vi "Add to Symbol Map.vi"(8 "error in (no error)":errorcluster, 9 ".NET Symbol Information":refnum<k24>, 10 "Symbol Name":string, 11 "TwinCAT ADS in":refnum<class "TwinCAT ADS.lvclass">) -> (0 "error out":errorcluster, 2 "Success?":bool, 3 "TwinCAT ADS out":refnum<class "TwinCAT ADS.lvclass">)   [LabVIEW 2018, in "TwinCAT ADS.lvclass"]
uses:
  TwinCAT ADS.lvclass
  TwinCAT.Ads
  TwinCAT ADS.lvclass/TwinCAT ADS.ctl
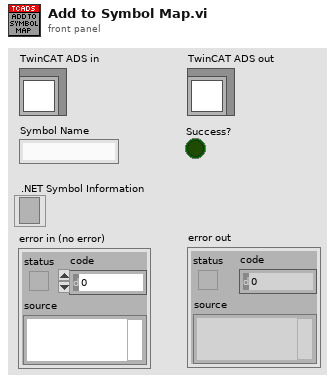
[diagram p1: front panel]
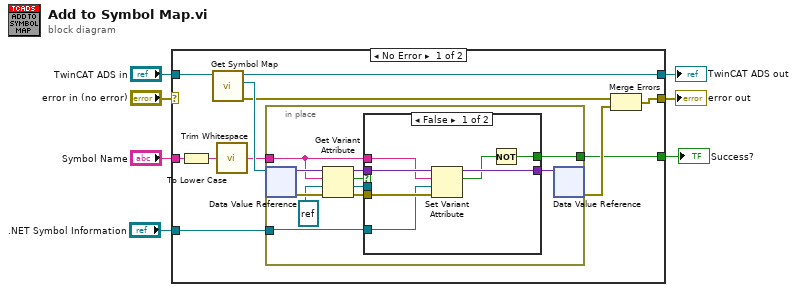
[diagram p0: block diagram]
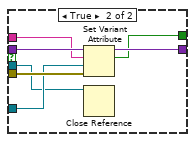
[diagram p2: hidden frame]
diagram:
  n1 = case shown="No Error" "error in (no error)" {
    selector: "error in (no error)" -> [_ w44]
    tunnel: "TwinCAT ADS in" -> [w18 w45]
    tunnel: ".NET Symbol Information" -> [w16 _]
    tunnel: "Symbol Name" -> [w15 _]
    tunnel: [w12 w45] -> w4
    tunnel: [w11 w44] -> w3
    tunnel: [w8 _] -> w1
    frame No Error {
      n2 = To Lower Case(string=w15) -> (all lower case string=w10:string)
      n3 = call "Get Symbol Map.vi"("TwinCAT ADS in"=w18) -> ("error out"=w14:errorcluster, "Symbol Map"=w17:refnum<data-value>, "TwinCAT ADS out"=w12:refnum<class "TwinCAT ADS.lvclass">)  [unwired: 8 in]
      n4 = call <vilib>:"Trim Whitespace.vi"("string"=w10) -> ("trimmed string"=w9:string)  [unwired: 1 in]
      n5 = in-place {
        in-place-border: w16 -> [w24]
        in-place-border: w9 -> [w23]
        in-place-border: [w19] -> w8
        n6 = in-place-dvr #1(w17) -> (w28:variant, w29:errorcluster)
        n7 = Get Variant Attribute(Variant=w28, name=w23, default value (empty Variant)=refnum<k24> refnum (".NET Symbol Information"), error in=w29) -> (duplicate Variant=w27:variant, found=w22:bool, value=w20:refnum<k24>, error out=w25:errorcluster)
        n8 = case shown="False" w22 {
          tunnel: w27 -> [w36 w41]
          tunnel: [w35 w40] -> w26
          tunnel: w25 -> [w34 w43]
          tunnel: w24 -> [w32 w42]
          tunnel: w23 -> [w33 w38]
          tunnel: w20 -> [_ w37]
          tunnel: [w30 w39] -> w19
          frame False {
            n9 = Set Variant Attribute(Variant=w36, name=w33, value=w32, error in=w34) -> (Variant out=w35:variant, replaced=w31:bool)  [unwired: 1 out]
            n10 = Not(x=w31) -> (.not. x?=w30:bool)
          }
          frame True {
            n11 = Set Variant Attribute(Variant=w41, name=w38, value=w42, error in=w43) -> (Variant out=w40:variant, replaced=w39:bool)  [unwired: 1 out]
            n12 = Close Reference(reference=w37) -> ()  [unwired: 1 in, 1 out]
          }
        }
        n13 = in-place-dvr #1(w26) -> (w13:errorcluster)  [unwired: 1 out]
      }
      n14 = Merge Errors(w14, w13) -> (w11:errorcluster)
    }
    frame Error {
    }
  }
  "error out" <- w3
  "TwinCAT ADS out" <- w4
  "Success?" <- w1
